vi "DMMs_terminate.vi"(8 "error in (no error)":errorcluster, 11 "DMMsData in":refnum<class "DMMsData.lvclass">) -> (0 "error out":errorcluster, 3 "DMMsData out":refnum<class "DMMsData.lvclass">)   [LabVIEW 2017, in "DMMsData.lvclass"]
uses:
  DMMsData.lvclass
  DMMsData.lvclass/DMMsData.ctl
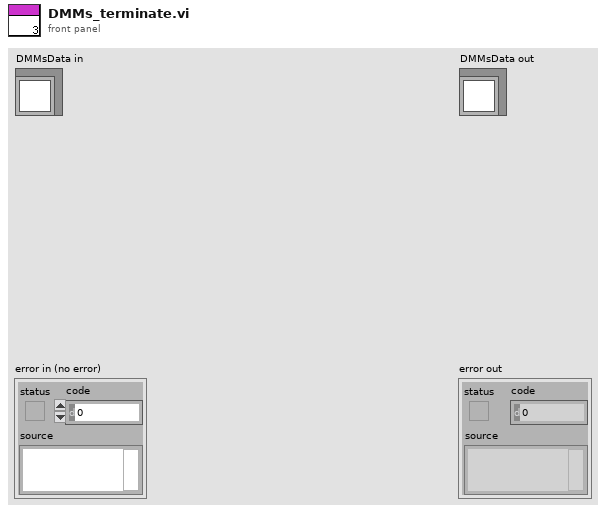
[diagram p1: front panel]
types:
  T1 = cluster{"Label":string, "Active?":bool, "VISA resource name":refnum<visa-resource-name>, "Device":enum16{"Agilent34401A", "ADCMT7351", "HP3478A"}, "Measurement":enum16{"DC Volts", "DC Currents", "2-Wire Resistance", "4-Wire Resistance"}, "FileFormat":string}[]
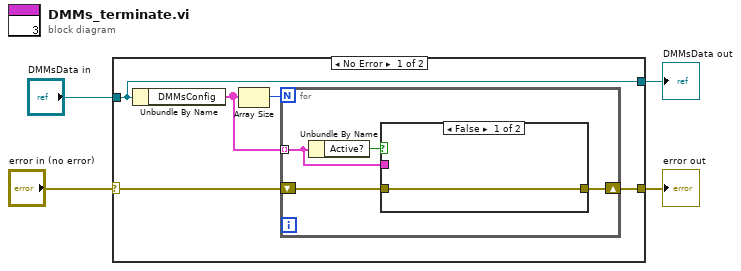
[diagram p0: block diagram]
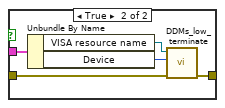
[diagram p2: hidden frame]
diagram:
  n1 = case shown="No Error" "error in (no error)" {
    selector: "error in (no error)" -> [w6 w21]
    tunnel: [w5 w21] -> w3
    tunnel: [w9 w20] -> w1
    tunnel: "DMMsData in" -> [w9 w20]
    frame No Error {
      n2 = Unbundle By Name(w9) -> ("DMMsConfig"=w7:T1)
      n3 = Array Size(array=w7) -> (size(s)=w8:i32)
      n4 = for {
        N: w8 -> [_]
        tunnel: w7 -> [w12] mode=indexing
        shift-right: [w10] -> w5
        shift-left: w6 -> [w11]
        n5 = Unbundle By Name(w12) -> ("Active?"=w13:bool)
        n6 = case shown="False" w13 {
          tunnel: w12 -> [_ w19]
          tunnel: w11 -> [w14 w16]
          tunnel: [w14 w15] -> w10
          frame False {
          }
          frame True {
            n7 = Unbundle By Name(w19) -> ("VISA resource name"=w18:refnum<visa-resource-name>, "Device"=w17:enum16{"Agilent34401A", "ADCMT7351", "HP3478A"})
            n8 = call "DDMs_low_terminate.vi"("error in (no error)"=w16, "Device"=w17, "VISA resource name"=w18) -> ("error out"=w15:errorcluster)  [unwired: 8 in]
          }
        }
      }
    }
    frame Error {
    }
  }
  "error out" <- w3
  "DMMsData out" <- w1
